vi "getNewImagePaths.vi"(8 "error in (no error)":errorcluster, 10 "numberOfImages":i32, 11 "FileNeologist in":refnum<class "FileNeologist.lvclass">) -> (0 "error out":errorcluster, 2 "Paths":path[](array[path]), 3 "FileNeologist out":refnum<class "FileNeologist.lvclass">)   [LabVIEW 2009, in "Tools.lvlib" / "Filing.lvlib" / "FileNeologist.lvclass"]
uses:
  FileNeologist.lvclass
  FileNeologist.lvclass/FileNeologist.ctl
panel:
  out "scriptName":string
  out "imagePaths":string[](array[string])
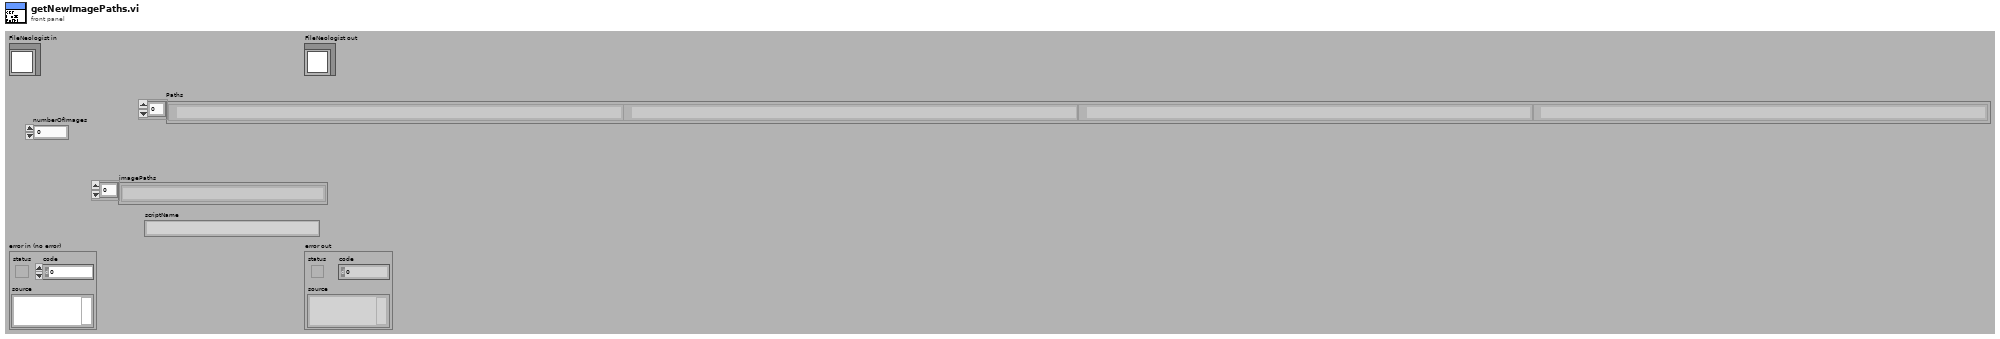
[diagram p1: front panel]
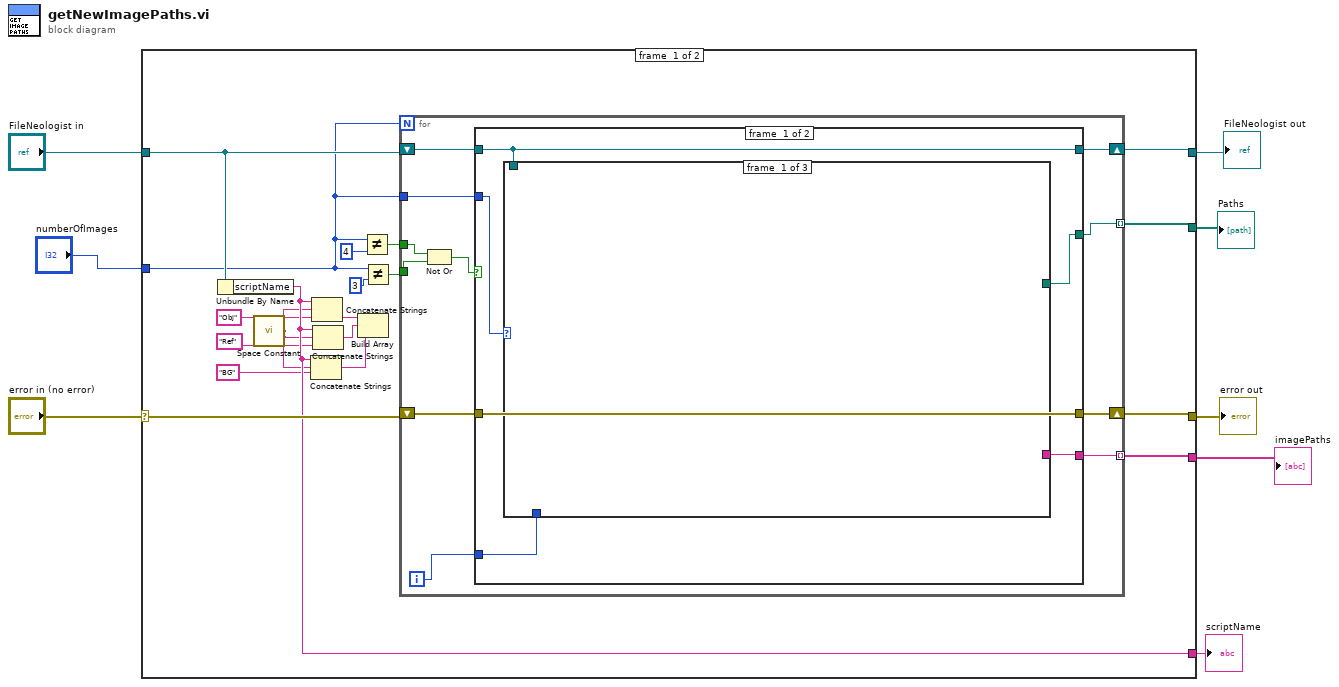
[diagram p0: block diagram]
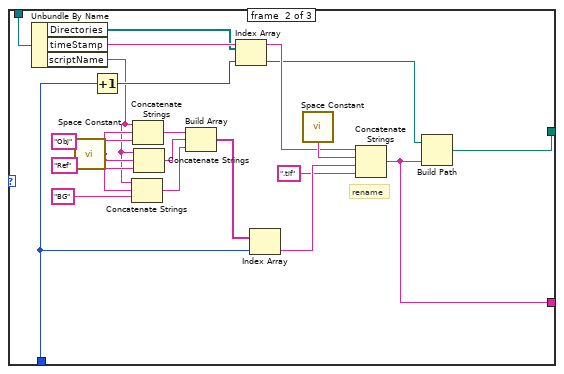
[diagram p2: hidden frame]
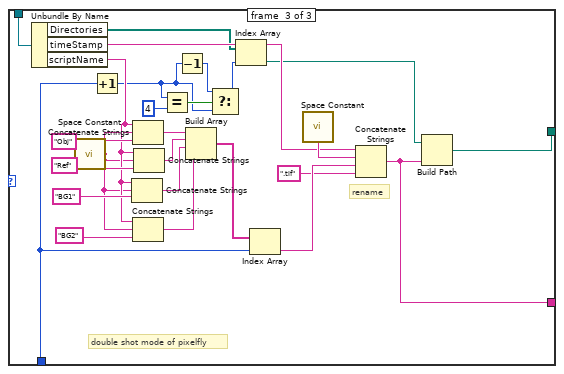
[diagram p3: hidden frame]
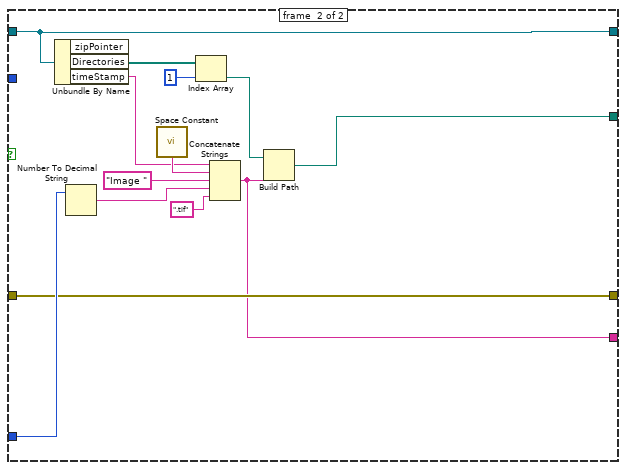
[diagram p4: hidden frame]
diagram:
  n1 = case shown="No Error" "error in (no error)" {
    selector: "error in (no error)" -> [w24 w105]
    tunnel: [w26 w105] -> w3
    tunnel: [w25 w104] -> w4
    tunnel: "FileNeologist in" -> [w23 w104]
    tunnel: [w27 _] -> w5
    tunnel: [w22 _] -> w1
    tunnel: [w21 _] -> w2
    tunnel: "numberOfImages" -> [w9 _]
    frame #0 {
      n2 = Unbundle By Name(w23) -> ("scriptName"=w22:string)
      n3 = call <vilib>:"Space Constant.vi"() -> ("String"=w14:string)
      n4 = Concatenate Strings(w22, w14, "BG") -> (w17:string)
      n5 = Concatenate Strings(w22, w14, "Obj") -> (w19:string)
      n6 = Concatenate Strings(w22, w14, "Ref") -> (w18:string)
      n7 = Build Array(w19, w18, w17) -> ()  [unwired: 1 out]
      n8 = Not Equal?(x=w9, y=4) -> (x != y?=w10:bool)
      n9 = Not Equal?(x=w9, y=3) -> (x != y?=w13:bool)
      n10 = for {
        N: w9 -> [_]
        tunnel: [w38] -> w27 mode=indexing
        shift-right: [w35] -> w25
        shift-left: w23 -> [w36]
        shift-right: [w37] -> w26
        shift-left: w24 -> [w34]
        tunnel: w13 -> [w30]
        tunnel: [w32] -> w21 mode=indexing
        tunnel: w10 -> [w31]
        tunnel: w9 -> [w28]
        i -> [w33]
        n11 = Not Or(1:w30, 2:w31) -> (0:w29:bool)
        n12 = case shown="True" w29 {
          tunnel: [w42 w94] -> w38
          tunnel: [w40 w92] -> w37
          tunnel: w36 -> [w41 w93]
          tunnel: [w41 w93] -> w35
          tunnel: w34 -> [w40 w92]
          tunnel: w33 -> [w44 w98]
          tunnel: [w43 w91] -> w32
          tunnel: w28 -> [w39 _]
          frame #0 {
            n13 = case shown="4" w39 {
              tunnel: w44 -> [_ w60 w86]
              tunnel: [_ w57 w84] -> w43
              tunnel: [_ w55 w82] -> w42
              tunnel: w41 -> [_ w54 w81]
              frame #0 {
              }
              frame #1 {
                # "rename"
                n14 = Unbundle By Name(w54) -> ("Directories"=w62:path[], "timeStamp"=w63:string, "scriptName"=w49:string)
                n15 = call <vilib>:"Space Constant.vi"() -> ("String"=w50:string)
                n16 = Increment(x=w60) -> (x+1=w59:i32)
                n17 = Concatenate Strings(w49, w50, "BG") -> (w47:string)
                n18 = Concatenate Strings(w49, w50, "Obj") -> (w48:string)
                n19 = Concatenate Strings(w49, w50, "Ref") -> (w46:string)
                n20 = Build Array(w48, w46, w47) -> (w45:string[])
                n21 = Index Array(array=w62, index=w59) -> (element=w61:path)
                n22 = Index Array(array=w45, index=w60) -> (element=w58:string)
                n23 = call <vilib>:"Space Constant.vi"() -> ("String"=w64:string)
                n24 = Concatenate Strings(w63, w64, w58, ".tif") -> (w57:string)
                n25 = Build Path(base path=w61, name or relative path=w57) -> (appended path=w55:path)
              }
              frame #2 {
                # "double shot mode of pixelfly"
                # "rename"
                n26 = Unbundle By Name(w81) -> ("Directories"=w88:path[], "timeStamp"=w89:string, "scriptName"=w73:string)
                n27 = call <vilib>:"Space Constant.vi"() -> ("String"=w72:string)
                n28 = Increment(x=w86) -> (x+1=w66:i32)
                n29 = Concatenate Strings(w73, w72, "BG1") -> (w76:string)
                n30 = Concatenate Strings(w73, w72, "Obj") -> (w77:string)
                n31 = Concatenate Strings(w73, w72, "BG2") -> (w70:string)
                n32 = Concatenate Strings(w73, w72, "Ref") -> (w75:string)
                n33 = Equal?(x=w66, y=4) -> (x = y?=w68:bool)
                n34 = Decrement(x=w66) -> (x-1=w67:i32)
                n35 = Build Array(w77, w75, w76, w70) -> (w74:string[])
                n36 = Select(t=w67, s=w68, f=w66) -> (s? t:f=w65:i32)
                n37 = Index Array(array=w88, index=w65) -> (element=w87:path)
                n38 = Index Array(array=w74, index=w86) -> (element=w85:string)
                n39 = call <vilib>:"Space Constant.vi"() -> ("String"=w90:string)
                n40 = Concatenate Strings(w89, w90, w85, ".tif") -> (w84:string)
                n41 = Build Path(base path=w87, name or relative path=w84) -> (appended path=w82:path)
              }
            }
          }
          frame #1 {
            n42 = Unbundle By Name(w93) -> ("Directories"=w101:path[], "timeStamp"=w102:string)  [unwired: 1 out]
            n43 = Number To Decimal String(number=w98) -> (decimal integer string=w96:string)  [unwired: 1 in]
            n44 = call <vilib>:"Space Constant.vi"() -> ("String"=w103:string)
            n45 = Index Array(array=w101, index=1) -> (element=w100:path)
            n46 = Concatenate Strings(w102, w103, "Image ", w96, ".tif") -> (w91:string)
            n47 = Build Path(base path=w100, name or relative path=w91) -> (appended path=w94:path)
          }
        }
      }
    }
    frame #1 {
    }
  }
  "error out" <- w3
  "FileNeologist out" <- w4
  "Paths" <- w5
  "imagePaths" <- w2
  "scriptName" <- w1
